vi "PWV_dPdU(SubVI).vi"(10 "Flow Velocity (m/s)":dbl[](array[numeric]), 11 "Pressure (mmHg)":dbl[](array[numeric])) -> (3 "PWV (m/s) (dPdU)":dbl=13.069900011809668)   [LabVIEW 2017]
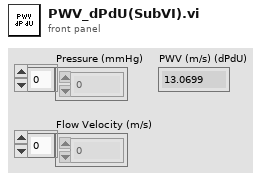
[diagram p1: front panel]
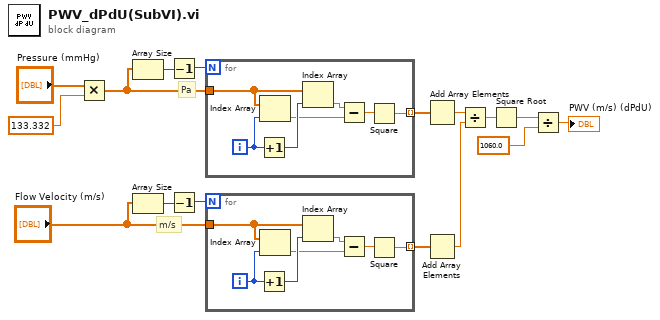
[diagram p0: block diagram]
diagram:
  # "m/s"
  # "Pa"
  n1 = Multiply(x="Pressure (mmHg)", y=133.332 ("x")) -> (x*y=w7:dbl[])
  n2 = Array Size(array=w7) -> (size(s)=w6:i32)
  n3 = Array Size(array="Flow Velocity (m/s)") -> (size(s)=w4:i32)
  n4 = Decrement(x=w6) -> (x-1=w5:i32)
  n5 = Decrement(x=w4) -> (x-1=w3:i32)
  n6 = for {
    N: w5 -> [_]
    tunnel: w7 -> [w21]
    tunnel: [w17] -> w8 mode=indexing
    i -> [w22]
    n7 = Increment(x=w22) -> (x+1=w23:i32)
    n8 = Index Array(array=w21, index=w22) -> (element=w19:dbl)
    n9 = Index Array(array=w21, index=w23) -> (element=w20:dbl)
    n10 = Subtract(x=w20, y=w19) -> (x-y=w18:dbl)
    n11 = Square(x=w18) -> (x^2=w17:dbl)
  }
  n12 = for {
    N: w3 -> [_]
    tunnel: "Flow Velocity (m/s)" -> [w28]
    tunnel: [w24] -> w9 mode=indexing
    i -> [w29]
    n13 = Increment(x=w29) -> (x+1=w30:i32)
    n14 = Index Array(array=w28, index=w29) -> (element=w26:dbl)
    n15 = Index Array(array=w28, index=w30) -> (element=w27:dbl)
    n16 = Subtract(x=w27, y=w26) -> (x-y=w25:dbl)
    n17 = Square(x=w25) -> (x^2=w24:dbl)
  }
  n18 = Add Array Elements(numeric array=w8) -> (sum=w10:dbl)
  n19 = Add Array Elements(numeric array=w9) -> (sum=w11:dbl)
  n20 = Divide(x=w10, y=w11) -> (x/y=w12:dbl)
  n21 = Square Root(x=w12) -> (sqrt(x)=w13:dbl)
  n22 = Divide(x=w13, y=1060.0 ("x")) -> (x/y=→"PWV (m/s) (dPdU)":dbl)
